vi "Config.vi"(8 "error in (no error)":errorcluster, 10 "Digital Configuration":T1) -> (0 "error out":errorcluster, 3 "TCP 380 out":refnum<class "TCP 380.lvclass">)   [LabVIEW 2021, in "TCP 380.lvlib" / "TCP 380.lvclass"]
uses:
  TCP 380.lvclass
  DAQ-arch/Digital Configure.ctl
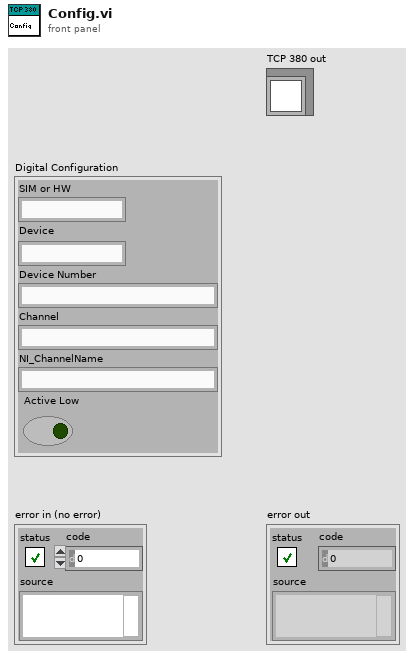
[diagram p1: front panel]
types:
  T1 = typedef "Digital Configure.ctl" = cluster{"SIM or HW":string, "Device":string, "Device Number":string, "Channel":string, "NI_ChannelName":string, "Active Low":bool}
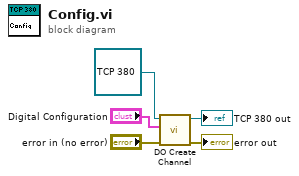
[diagram p0: block diagram]
diagram:
  n1 = call "DO Create Channel.vi"("error in (no error)"="error in (no error)", "Digital Configuration"="Digital Configuration", "TCP 380 in"=refnum<class "TCP 380.lvclass"> refnum) -> ("error out"=→"error out":errorcluster, "TCP 380 out"=→"TCP 380 out":refnum<class "TCP 380.lvclass">)  [unwired: 7 in]
